vi "parse_string.vi"   [LabVIEW 2012]
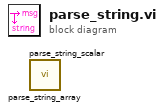
[diagram p0: block diagram]
diagram:
  n1 = call "parse_string_array.vi"() -> ()  [unwired: 5 in, 3 out]
  n2 = call "parse_string_scalar.vi"() -> ()  [unwired: 5 in, 3 out]
